vi "Set Speed.vi"(8 "error in (no error)":errorcluster, 10 "speed":dbl, 11 "VICI Settings In":T1 {"Pump Number" min=0.0 max=20.0 step=1.0}) -> (0 "error out":errorcluster, 1 "Connection Error":bool, 3 "VICI Settings Out":T1 {"Pump Number" min=0.0 max=20.0 step=1.0})   [LabVIEW 2018, in "VICI M50.lvlib"]
uses:
  VICI M50.lvlib
  Settings Cluster.ctl
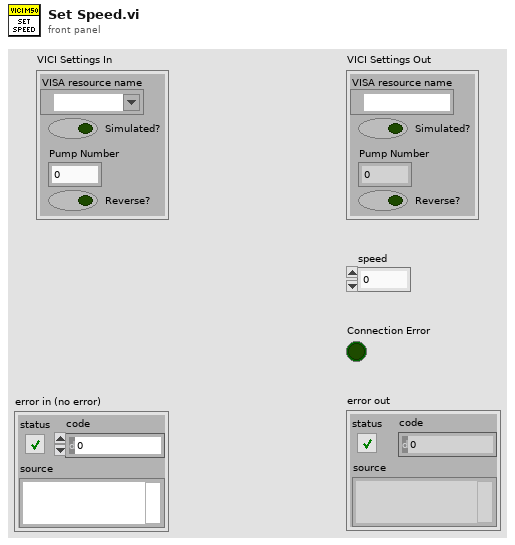
[diagram p1: front panel]
types:
  T1 = typedef "Settings Cluster.ctl" = cluster{"VISA resource name":refnum<visa-resource-name>, "Simulated?":bool, "Pump Number":dbl, "Reverse?":bool}
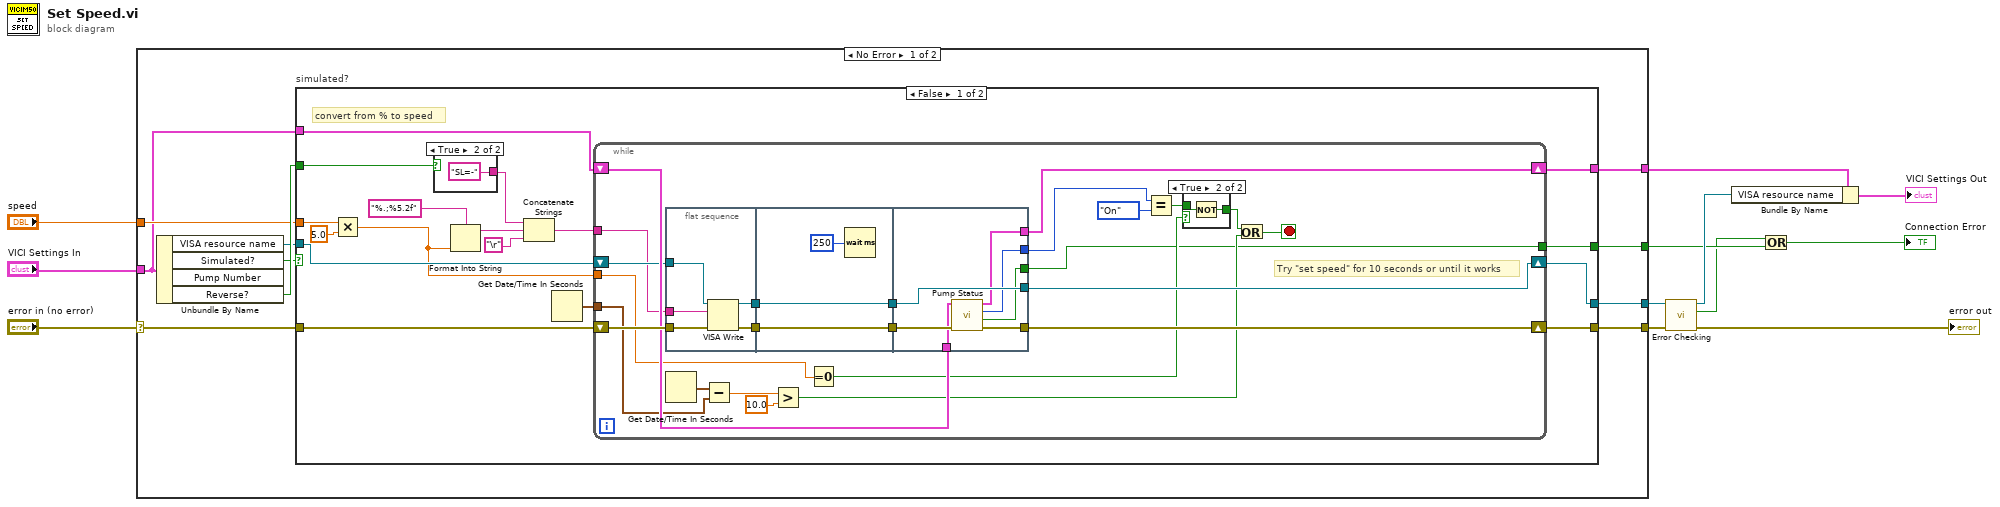
[diagram p0: block diagram]
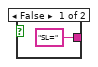
[diagram p3: hidden frame]
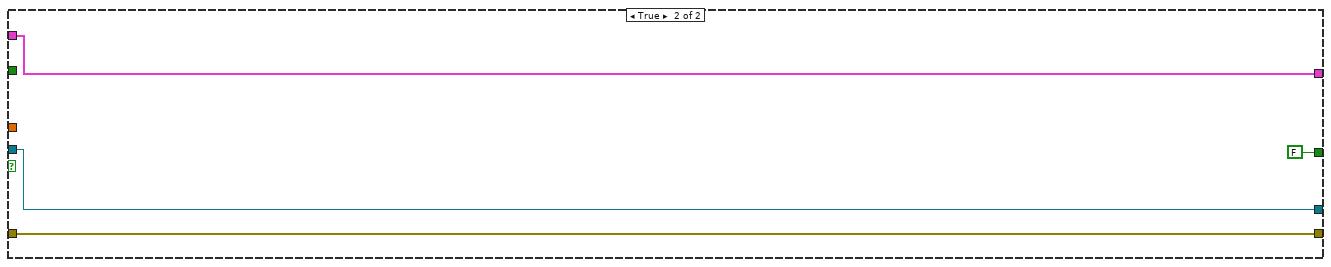
[diagram p4: hidden frame]
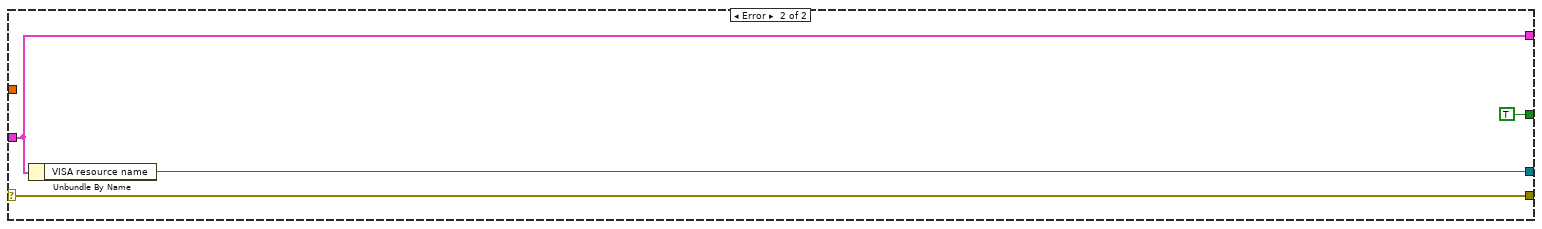
[diagram p5: hidden frame]
diagram:
  n1 = case shown="No Error" "error in (no error)" {
    selector: "error in (no error)" -> [w19 w91]
    tunnel: [w14 w90] -> w5
    tunnel: "VICI Settings In" -> [w15 w90]
    tunnel: "speed" -> [w18 _]
    tunnel: [w17 w89] -> w9
    tunnel: [w16 w91] -> w8
    tunnel: [w13 TRUE ("Connection Error")] -> w3
    frame No Error {
      n2 = Unbundle By Name(w15) -> ("VISA resource name"=w21:refnum<visa-resource-name>, "Simulated?"=w20:bool, "Reverse?"=w22:bool)  [unwired: 1 out]
      n3 = case "simulated?" shown="False" w20 {
        tunnel: [w37 w87] -> w17
        tunnel: w21 -> [w39 w87]
        tunnel: w19 -> [w38 w86]
        tunnel: [w36 w86] -> w16
        tunnel: w22 -> [w35 _]
        tunnel: w18 -> [w33 _]
        tunnel: w15 -> [w31 w85]
        tunnel: [w30 w85] -> w14
        tunnel: [w27 FALSE ("Connection Error")] -> w13
        frame False {
          # "convert from % to speed"
          n4 = Multiply(x=w33, y=5.0) -> (x*y=w29:dbl)
          n5 = case shown="True" w35 {
            tunnel: ["SL=" ("string") "SL=-" ("string")] -> w26
            frame False {
            }
            frame True {
            }
          }
          n6 = Format Into String(format string="%.;%5.2f", w29) -> (resulting string=w25:string)  [unwired: 2 in, 1 out]
          n7 = Concatenate Strings(w26, w25, "\r") -> (w24:string)
          n8 = Get Date/Time In Seconds() -> (seconds since 1Jan1904=w28:timestamp)
          n9 = while {
            shift-right: [w58] -> w37
            shift-left: w39 -> [w45]
            shift-right: [w57] -> w36
            shift-left: w38 -> [w59]
            shift-right: [w55] -> w30
            shift-left: w31 -> [w56]
            tunnel: w29 -> [w54]
            tunnel: w28 -> [w47]
            tunnel: [w44] -> w27
            tunnel: w24 -> [w40]
            stop <- w50 stop-if-true
            # "Try \"set speed\" for 10 seconds or until it works"
            n10 = flat-sequence {
              tunnel: w45 -> [w71]
              tunnel: w59 -> [w70]
              tunnel: [w69] -> w63
              tunnel: [w68] -> w62
              tunnel: w40 -> [w67]
              tunnel: w63 -> [w74]
              tunnel: w62 -> [w73]
              tunnel: [w74] -> w61
              tunnel: [w73] -> w60
              tunnel: [w79] -> w57
              tunnel: [w81] -> w58
              tunnel: w61 -> [w81]
              tunnel: w60 -> [w80]
              tunnel: w56 -> [w78]
              tunnel: [w77] -> w55
              tunnel: [w76] -> w43
              tunnel: [w75] -> w44
              frame #0 {
                n11 = VISA Write(VISA resource name=w71, write buffer=w67, error in (no error)=w70) -> (VISA resource name out=w69:refnum<visa-resource-name>, error out=w68:errorcluster)  [unwired: 1 out]
              }
              frame #1 {
                n12 = Wait (ms)(milliseconds to wait=u32 250) -> ()  [unwired: 1 out]
              }
              frame #2 {
                n13 = call "Pump Status.vi"("error in (no error)"=w80, "VICI Settings In"=w78) -> ("error out"=w79:errorcluster, "Connection Error"=w75:bool, "Pump On?"=w76:enum16{"Off", "On", "Not Initialized"}, "VICI Settings Out"=w77:T1)  [unwired: 6 in]
              }
            }
            n14 = Get Date/Time In Seconds() -> (seconds since 1Jan1904=w46:timestamp)
            n15 = Subtract(x=w46, y=w47) -> (x-y=w52:dbl)
            n16 = Greater?(x=w52, y=10.0) -> (0:w48:bool)
            n17 = Equal To 0?(x=w54) -> (x = 0?=w53:bool)
            n18 = Equal?(x=w43, y=enum16{"Off", "On", "Not Initialized"}."On") -> (x = y?=w42:bool)
            n19 = case shown="True" w53 {
              tunnel: [w64 w66] -> w51
              tunnel: w42 -> [w64 w65]
              frame False {
              }
              frame True {
                n20 = Not(x=w65) -> (.not. x?=w66:bool)
              }
            }
            n21 = Or(x=w51, y=w48) -> (x .or. y?=w50:bool)
          }
        }
        frame True {
        }
      }
    }
    frame Error {
      n22 = Unbundle By Name(w90) -> ("VISA resource name"=w89:refnum<visa-resource-name>)
    }
  }
  n23 = call "Error Checking.vi"("error in (no error)"=w8, "VISA resource name"=w9) -> ("error out"=→"error out":errorcluster, "Connection Error"=w2:bool, "VISA resource name"=w6:refnum<visa-resource-name>)  [unwired: 7 in]
  n24 = Bundle By Name(cluster=w5, "VISA resource name"=w6) -> (→"VICI Settings Out":T1)
  n25 = Or(x=w2, y=w3) -> (x .or. y?=→"Connection Error":bool)
